vi "auto_sub_vi.vi"(11 "디지털 입력":refnum<vi>) -> ()   [LabVIEW 2020]
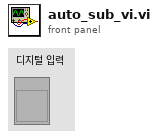
[diagram p1: front panel]
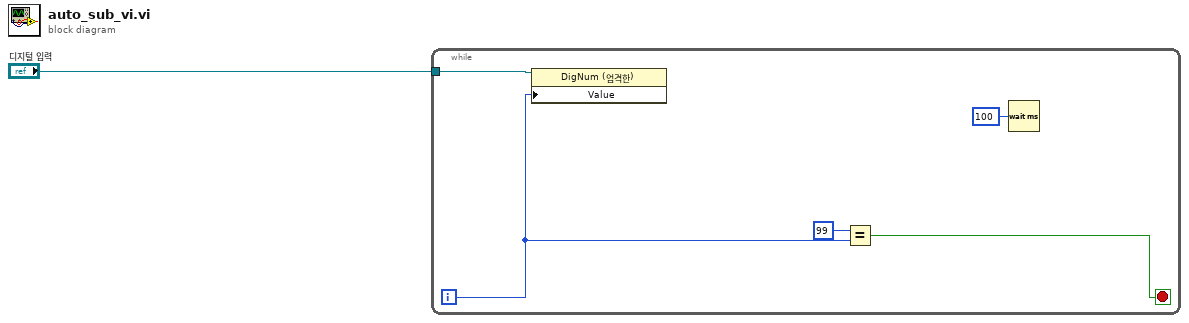
[diagram p0: block diagram]
diagram:
  n1 = while {
    tunnel: "디지털 입력" -> [w6]
    i -> [w4]
    stop <- w2 stop-if-true
    n2 = property class="DigNum (엄격한)"(reference=w6, "Value"=w4) -> ()  [unwired: 1 in, 2 out]
    n3 = Equal?(x=99, y=w4) -> (x = y?=w2:bool)
    n4 = Wait (ms)(milliseconds to wait=u32 100 ("대기 시간 (ms)")) -> ()  [unwired: 1 out]
  }
